vi "EdgeDetect.vi"() -> ()   [LabVIEW 2019]
uses:
  <vilib>/vision/Measure.llb/Edge New.ctl
  <vilib>/userDefined/High Color/IMAQdx.ctl
  <vilib>/vision/driver/NI_Vision_Acquisition_Software.lvlib
  <vilib>/vision/NI_Vision_Development_Module.lvlib
panel:
  out "Edge Information":T1[](array[typedef]) {"Distance (Real-World)" format="%.2f"; "Location (Real-World)"."Y" format="%.2g"; "Location (Real-World)"."X" format="%.2f"; "Noise" format="%.2f"; "Location (Pixel)"."Y" format="%.2g"; "Location (Pixel)"."X" format="%.2f"; "Strength" format="%.2f"; "Distance (Pixel)" format="%.2f"}
  out "Straight Edges":T2(array[cluster]) {"Point2 (Real-World)"."Y" format="%.2f"; "Point2 (Real-World)"."X" format="%.2f"; "Point1 (Real-World)"."Y" format="%.2f"; "Point1 (Real-World)"."X" format="%.2f"; "Point2 (Pixels)"."Y" format="%.2f"; "Point2 (Pixels)"."X" format="%.2f"; "Point1 (Pixels)"."Y" format="%.2f"; "Point1 (Pixels)"."X" format="%.2f"}
  out "error out":errorcluster
  in  "Circle Descriptor":cluster{"Min Radius":dbl, "Max Radius":dbl}={"Min Radius"=90.0, "Max Radius"=500.0}
  out "Number of Matches Returned":i32
  out "Circles":T3(array[cluster]) {"Position"."Y" format="%.2f"; "Position"."X" format="%.2f"}
  in  "Image Type":T4 items=["Grayscale (U8)", "Grayscale (I16)", "Grayscale (SGL)", "Complex (CSG)", "RGB (U32)", "HSL (U32)", "RGB (U64)", "Grayscale (U16)"]
  out "Image 2":T5(plugin-control)
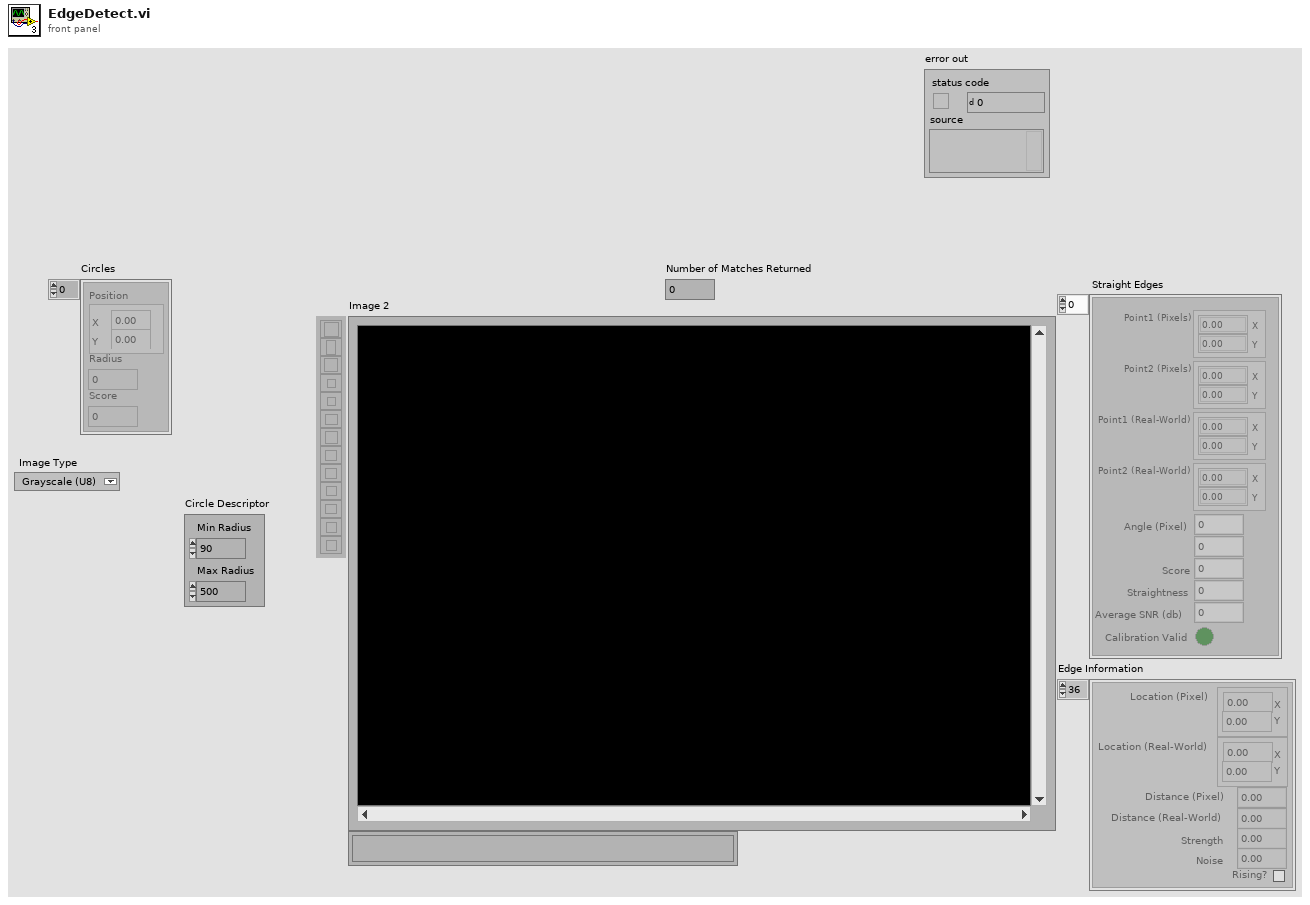
[diagram p1: front panel]
types:
  T1 = typedef "Edge New.ctl" = cluster{"Location (Pixel)":cluster{"X":sgl, "Y":sgl}, "Location (Real-World)":cluster{"X":sgl, "Y":sgl}, "Distance (Pixel)":dbl, "Distance (Real-World)":dbl, "Strength":dbl, "Noise":dbl, "Rising?":bool}
  T2 = cluster{"Point1 (Pixels)":cluster{"X":sgl, "Y":sgl}, "Point2 (Pixels)":cluster{"X":sgl, "Y":sgl}, "Point1 (Real-World)":cluster{"X":sgl, "Y":sgl}, "Point2 (Real-World)":cluster{"X":sgl, "Y":sgl}, "Angle (Pixel)":dbl, "Angle (Real-World)":dbl, "Score":dbl, "Straightness":dbl, "Average SNR (db)":dbl, "Calibration Valid":bool}[]
  T3 = cluster{"Position":cluster{"X":sgl, "Y":sgl}, "Radius":dbl, "Score":dbl}[]
  T4 = typedef "Image Type" = u32
  T5 = typedef "IMAQ Image.ctl" = refnum<image>
  T6 = typedef "IMAQ Rectangle" = cluster{"Left":i32, "Top":i32, "Right":i32, "Bottom":i32, "Rotation":dbl}
  T7 = typedef "IMAQ Circle" = cluster{"Center X":i32, "Center Y":i32, "Inner Radius":i32, "Outer Radius":i32, "Start Angle":dbl, "End Angle":dbl}
  T8 = typedef "IMAQdx.ctl" = refnum<k21>
  T9 = typedef "ROI Descriptor" = cluster{"Global Rectangle":i32[], "Contours":cluster{"ID":enum32{"External", "Internal"}, "Type":u32, "Coordinates":i32[]}[]}
  T10 = cluster{"Circles[0]":cluster{"Position":cluster{"X":sgl, "Y":sgl}, "Radius":dbl, "Score":dbl}, "Circles[1]":cluster{"Position":cluster{"X":sgl, "Y":sgl}, "Radius":dbl, "Score":dbl}, "Circles[2]":cluster{"Position":cluster{"X":sgl, "Y":sgl}, "Radius":dbl, "Score":dbl}, "Circles[3]":cluster{"Position":cluster{"X":sgl, "Y":sgl}, "Radius":dbl, "Score":dbl}, "Circles[4]":cluster{"Position":cluster{"X":sgl, "Y":sgl}, "Radius":dbl, "Score":dbl}, "Circles[5]":cluster{"Position":cluster{"X":sgl, "Y":sgl}, "Radius":dbl, "Score":dbl}, "Circles[6]":cluster{"Position":cluster{"X":sgl, "Y":sgl}, "Radius":dbl, "Score":dbl}, "Circles[7]":cluster{"Position":cluster{"X":sgl, "Y":sgl}, "Radius":dbl, "Score":dbl}, "Circles[8]":cluster{"Position":cluster{"X":sgl, "Y":sgl}, "Radius":dbl, "Score":dbl}}
  T11 = cluster{"Position":cluster{"X":sgl, "Y":sgl}, "Radius":dbl, "Score":dbl}
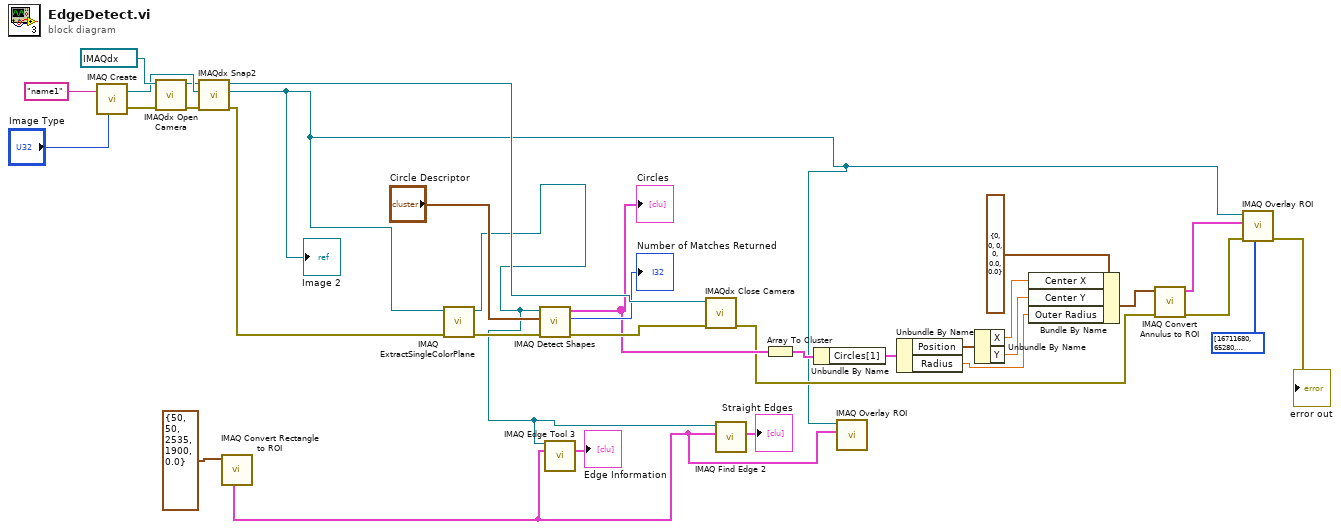
[diagram p0: block diagram]
diagram:
  n1 = call "IMAQ Create"("Image Name"="name1", "Image Type"="Image Type") -> ("New Image"=w30:T5, "error out"=w27:errorcluster)  [unwired: 3 in]
  n2 = call <vilib>:"IMAQdx Open Camera.vi"("error in"=w27, "Session In"=T8 "cam0") -> ("error out"=w31:errorcluster, "Session Out"=w29:T8)  [unwired: 8 in]
  n3 = call <vilib>:"IMAQdx Snap2.vi"("error in"=w31, "Image In"=w30, "Session In"=w29) -> ("error out"=w24:errorcluster, "Image Out"=w5:T5, "Session Out"=w28:T8)  [unwired: 6 in]
  "Image 2" <- w5
  n4 = call "IMAQ Convert Rectangle to ROI"("Rectangle"=T6 {"Left"=50, "Top"=50, "Right"=2535, "Bottom"=1900, "Rotation"=0.0}) -> ("ROI Descriptor"=w2:T9)  [unwired: 8 in, 1 out]
  n5 = call "IMAQ ExtractSingleColorPlane"("error in (no error)"=w24, "Image Src"=w5) -> ("error out"=w23:errorcluster, "Image Dst Out"=w3:T5)  [unwired: 2 in, 6 out]
  n6 = call-poly "IMAQ Detect Shapes"("error in (no error)"=w23, "Circle Descriptor"="Circle Descriptor", "Image"=w3) -> ("error out"=w25:errorcluster, "Number of Matches Returned"=→"Number of Matches Returned":i32, "Circles"=w14:T3)  [unwired: 4 in, 2 out]
  "Circles" <- w14
  n7 = call "IMAQ Edge Tool 3"("Image"=w3, "ROI Descriptor"=w2) -> ("Edge Information"=→"Edge Information":T1[])  [unwired: 9 in, 4 out]
  n8 = call <vilib>:"IMAQdx Close Camera.vi"("error in"=w25, "Session In"=w28) -> ("error out"=w11:errorcluster)  [unwired: 9 in]
  n9 = call "IMAQ Find Edge 2"("ROI Descriptor"=w2, "Image"=w3) -> ("Straight Edges"=→"Straight Edges":T2)  [unwired: 6 in, 3 out]
  n10 = Array To Cluster(array=w14) -> (cluster=w13:T10)
  n11 = Unbundle By Name(w13) -> ("Circles[1]"=w12:T11)
  n12 = call "IMAQ Overlay ROI"("ROI Descriptor"=w2, "Image"=w5) -> ()  [unwired: 8 in, 2 out]
  n13 = Unbundle By Name(w12) -> ("Position"=w18:cluster{"X":sgl, "Y":sgl}, "Radius"=w15:dbl)
  n14 = Unbundle By Name(w18) -> ("X"=w17:sgl, "Y"=w16:sgl)
  n15 = Bundle By Name(cluster=T7 {"Center X"=0, "Center Y"=0, "Inner Radius"=0, "Outer Radius"=0, "Start Angle"=0.0, "End Angle"=0.0} ("Annulus"), "Center X"=w17, "Center Y"=w16, "Outer Radius"=w15) -> (w20:T7)
  n16 = call "IMAQ Convert Annulus to ROI"("error in (no error)"=w11, "Annulus"=w20) -> ("error out"=w9:errorcluster, "ROI Descriptor"=w10:T9)  [unwired: 7 in]
  n17 = call "IMAQ Overlay ROI"("Colors (Green)"=u32[] [16711680, 65280, 2626303], "error in (no error)"=w9, "ROI Descriptor"=w10, "Image"=w5) -> ("error out"=→"error out":errorcluster)  [unwired: 6 in, 1 out]
